vi "Aspect Ratio Score.vi"(10 "Height":dbl, 11 "Width":dbl) -> (3 "Score":dbl)   [LabVIEW 2011]
doc: "Compare the ratio of the rectangle to that of the expected target. Score is in percent.\n\nSince inputs are particle measurements, the diagram doesn't expect to receive zero or negative values for either input."
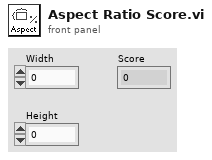
[diagram p1: front panel]
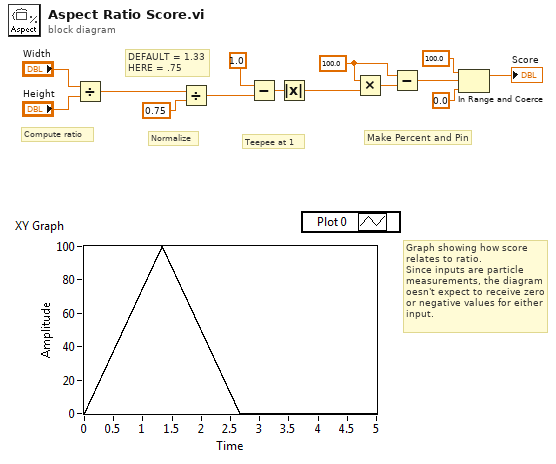
[diagram p0: block diagram]
diagram:
  w7 = 100.0 ("x/y")
  # "DEFAULT = 1.33\nHERE = .75"
  # "Graph showing how score\nrelates to ratio.\nSince inputs are particle\nmeasurements, the diagram\noesn't expect to receive zero\nor negative values for either\ninput."
  # "Make Percent and Pin"
  # "Teepee at 1"
  # "Normalize"
  # "Compute ratio"
  n1 = Divide(x="Width", y="Height") -> (x/y=w11:dbl)
  n2 = Divide(x=w11, y=0.75) -> (x/y=w9:dbl)
  n3 = Subtract(x=1.0 ("y"), y=w9) -> (x-y=w5:dbl)
  n4 = Absolute Value(x=w5) -> (abs(x)=w8:dbl)
  n5 = Multiply(x=w7, y=w8) -> (x*y=w10:dbl)
  n6 = Subtract(x=w7, y=w10) -> (x-y=w4:dbl)
  n7 = In Range and Coerce(upper limit=100.0, x=w4, lower limit=0.0) -> (coerced(x)=→"Score":dbl)  [unwired: 1 out]
